vi "StandardInit.vi"(1 "Incoming Handle":i32) -> (0 "Outgoing Handle":i32)   [LabVIEW 2011]
uses:
  Program Files (x86)/Gelles Lab Software/Madlib.dll
panel:
  out "Serial #":i32
  out "Aux axis":bool
  out "Aux Calibration":dbl format="%.3f"
  out "Z axis":bool
  out "Z Calibration":dbl format="%.3f"
  out "Y axis":bool
  out "Y Calibration":dbl format="%.3f"
  out "X axis":bool
  out "X Calibration":dbl caption="Calibration (um)" format="%.3f"
  out "DAC Freq (ms)":dbl format="%.4f"
  out "ADC Freq (ms)":dbl format="%.4f"
  out "Dll Revision":i16
  out "Dll Version":i16
  out "ADC resolution (bits)":i16
  out "DAC resolution (bits)":i16
  out "Product ID (in hex)":string
  out "Firmware Version":i16
  out "Firmware Profile":i16
  # "This VI implements an initialization sequence for use with \na single Nano-Drive."
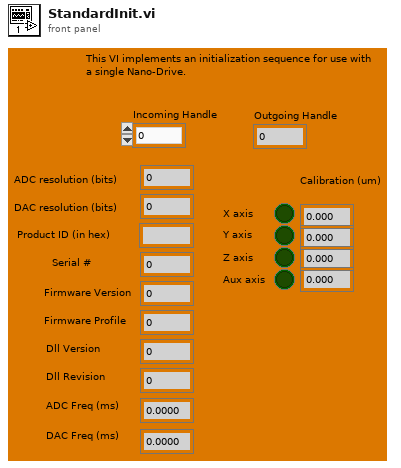
[diagram p1: front panel]
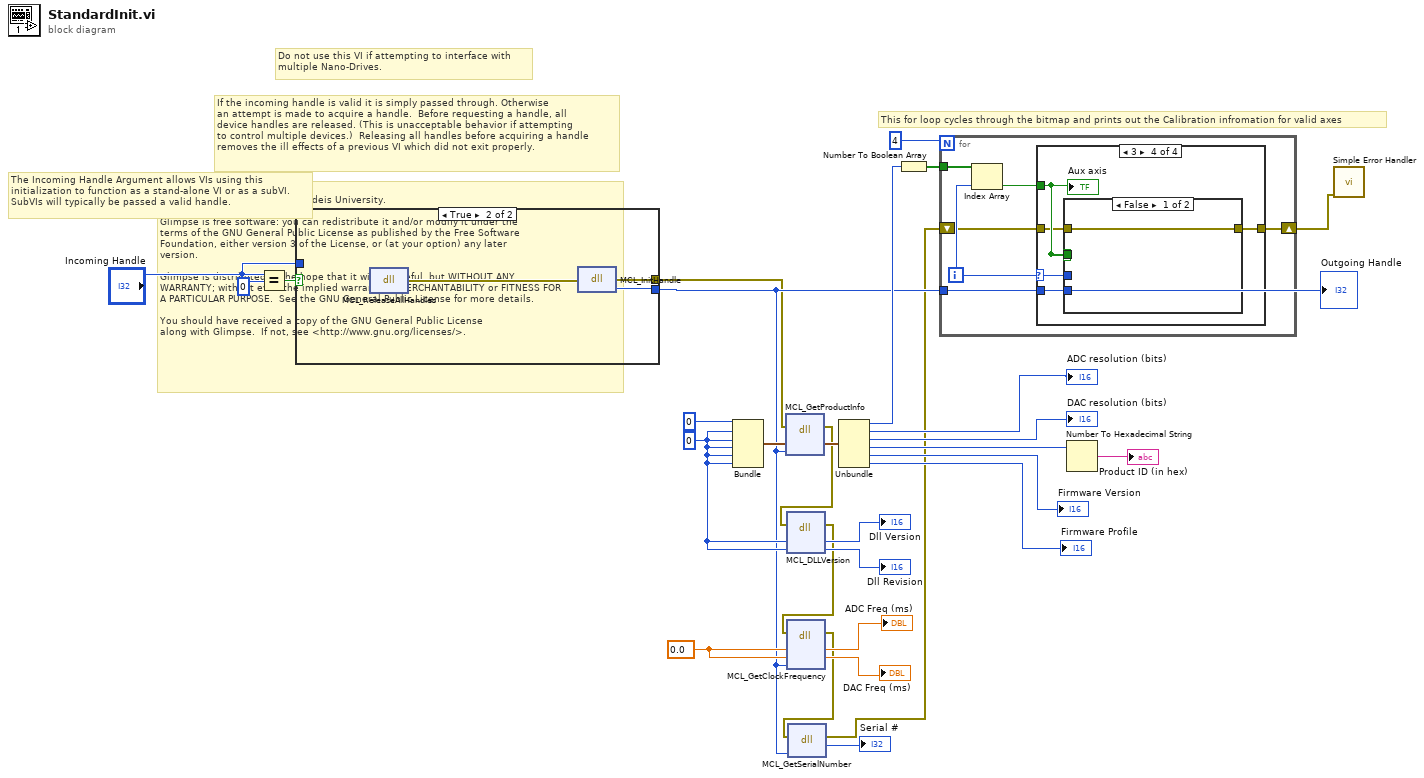
[diagram p0: block diagram]
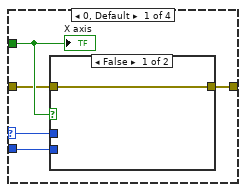
[diagram p2: hidden frame]
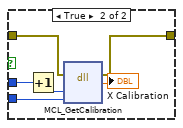
[diagram p3: hidden frame]
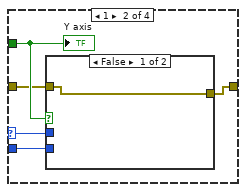
[diagram p4: hidden frame]
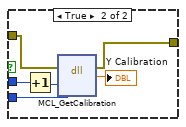
[diagram p5: hidden frame]
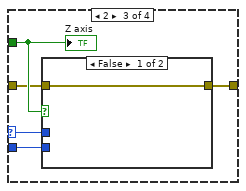
[diagram p6: hidden frame]
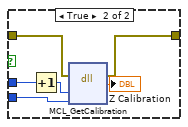
[diagram p7: hidden frame]
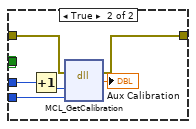
[diagram p8: hidden frame]
diagram:
  w14 = 0.0
  w17 = i16 0
  # "This file is part of Glimpse. \nCopyright 2014 Jeff Gelles, Brandeis University.    \n\nGlimpse is free software: you can redistribute it and/or modify it under the \nterms of the GNU General Public License as published by the Free Software \nFoundation, either version 3 of the License, or (at your option) any later \nversion.\n\nGlimpse is distributed in the hope that it will be useful, but WITHOUT ANY \nWARRANTY; without even the implied warranty of MERCHANTABILITY or FITNESS FOR \nA PARTICULAR PURPOSE.  See the GNU General Public License for more details.\n\nYou should have received a copy of the GNU General Public License\nalong with Glimpse.  If not, see <http://www.gnu.org/licenses/>."
  # "This for loop cycles through the bitmap and prints out the Calibration infromation for valid axes"
  # "The Incoming Handle Argument allows VIs using this\ninitialization to function as a stand-alone VI or as a subVI.\nSubVIs will typically be passed a valid handle."
  # "Do not use this VI if attempting to interface with\nmultiple Nano-Drives."
  # "If the incoming handle is valid it is simply passed through. Otherwise\nan attempt is made to acquire a handle.  Before requesting a handle, all\ndevice handles are released. (This is unacceptable behavior if attempting\nto control multiple devices.)  Releasing all handles before acquiring a handle\nremoves the ill effects of a previous VI which did not exit properly."
  n1 = Equal?(x="Incoming Handle", y=0) -> (x = y?=w28:bool)
  n2 = case shown="True" w28 {
    tunnel: [w30 w33] -> w7
    tunnel: "Incoming Handle" -> [w30 _]
    tunnel: [_ w31] -> w6
    frame False {
    }
    frame True {
      n3 = dll-call lib="C:/Program Files (x86)/Gelles Lab Software/MADLib.dll" fn="MCL_ReleaseAllHandles"() -> (error out=w32:errorcluster)  [unwired: 4 in, 1 out]
      n4 = dll-call lib="C:/Program Files (x86)/Gelles Lab Software/MADLib.dll" fn="MCL_InitHandle"(error in=w32) -> (error out=w31:errorcluster, "return type"=w33:i32)  [unwired: 2 in, 1 out]
    }
  }
  "Outgoing Handle" <- w7
  n5 = Bundle(u8 0, w17, w17, w17, w17, w17) -> (w25:cluster{u8, i16, i16, i16, i16, i16})  [unwired: 1 in]
  n6 = dll-call lib="C:/Program Files (x86)/Gelles Lab Software/MADLib.dll" fn="MCL_GetProductInfo"(error in=w6, w25, "handle"=w7) -> (error out=w5:errorcluster, w24:cluster{u8, i16, i16, i16, i16, i16})  [unwired: 4 in, 1 out]
  n7 = dll-call lib="C:/Program Files (x86)/Gelles Lab Software/MADLib.dll" fn="MCL_DLLVersion"(error in=w5, "version"=w17, "revision"=w17) -> (error out=w4:errorcluster, "version"=→"Dll Version":i16, "revision"=→"Dll Revision":i16)  [unwired: 3 in, 1 out]
  n8 = dll-call lib="C:/Program Files (x86)/Gelles Lab Software/MADLib.dll" fn="MCL_GetClockFrequency"(error in=w4, "ADC freq"=w14, "DAC freq"=w14, "handle"=w7) -> (error out=w3:errorcluster, "ADC freq"=→"ADC Freq (ms)":dbl, "DAC freq"=→"DAC Freq (ms)":dbl)  [unwired: 4 in, 1 out]
  n9 = dll-call lib="C:/Program Files (x86)/Gelles Lab Software/MADLib.dll" fn="MCL_GetSerialNumber"(error in=w3, "handle"=w7) -> (error out=w2:errorcluster, →"Serial #":i32)  [unwired: 3 in, 1 out]
  n10 = Unbundle(w24) -> (w11:u8, →"ADC resolution (bits)":i16, →"DAC resolution (bits)":i16, w23:i16, →"Firmware Version":i16, →"Firmware Profile":i16)
  n11 = Number To Boolean Array(number=w11) -> (Boolean array=w10:bool[])
  n12 = for {
    N: 4 -> [_]
    tunnel: w10 -> [w39]
    tunnel: w7 -> [w36]
    shift-right: [w34] -> w1
    shift-left: w2 -> [w35]
    i -> [w38]
    n13 = Index Array(array=w39, index=w38) -> (element=w37:bool)
    n14 = case shown="3" w38 {
      selector: w38 -> [w44 w56 w68 w80]
      tunnel: w37 -> [w43 w55 w67 w79]
      tunnel: w36 -> [w42 w54 w66 w78]
      tunnel: w35 -> [w41 w53 w65 w77]
      tunnel: [w40 w52 w64 w76] -> w34
      frame 0, Default {
        n15 = case shown="False" w43 {
          tunnel: w44 -> [_ w51]
          tunnel: w42 -> [_ w48]
          tunnel: w41 -> [w45 w47]
          tunnel: [w45 w46] -> w40
          frame False {
          }
          frame True {
            n16 = Increment(x=w51) -> (x+1=w49:i32)
            n17 = dll-call lib="C:/Program Files (x86)/Gelles Lab Software/MADLib.dll" fn="MCL_GetCalibration"(error in=w47, "axis"=w49, "handle"=w48) -> (error out=w46:errorcluster, →"X Calibration":dbl)  [unwired: 4 in, 1 out]
          }
        }
        "X axis" <- w43
      }
      frame 1 {
        n18 = case shown="False" w55 {
          tunnel: w56 -> [_ w63]
          tunnel: w54 -> [_ w61]
          tunnel: w53 -> [w57 w59]
          tunnel: [w57 w58] -> w52
          frame False {
          }
          frame True {
            n19 = Increment(x=w63) -> (x+1=w62:i32)
            n20 = dll-call lib="C:/Program Files (x86)/Gelles Lab Software/MADLib.dll" fn="MCL_GetCalibration"(error in=w59, "axis"=w62, "handle"=w61) -> (error out=w58:errorcluster, →"Y Calibration":dbl)  [unwired: 4 in, 1 out]
          }
        }
        "Y axis" <- w55
      }
      frame 2 {
        n21 = case shown="False" w67 {
          tunnel: w68 -> [_ w75]
          tunnel: w66 -> [_ w73]
          tunnel: w65 -> [w69 w71]
          tunnel: [w69 w70] -> w64
          frame False {
          }
          frame True {
            n22 = Increment(x=w75) -> (x+1=w72:i32)
            n23 = dll-call lib="C:/Program Files (x86)/Gelles Lab Software/MADLib.dll" fn="MCL_GetCalibration"(error in=w71, "axis"=w72, "handle"=w73) -> (error out=w70:errorcluster, →"Z Calibration":dbl)  [unwired: 4 in, 1 out]
          }
        }
        "Z axis" <- w67
      }
      frame 3 {
        n24 = case shown="False" w79 {
          tunnel: w80 -> [_ w87]
          tunnel: w79 -> [_ _]
          tunnel: w78 -> [_ w84]
          tunnel: w77 -> [w81 w83]
          tunnel: [w81 w82] -> w76
          frame False {
          }
          frame True {
            n25 = Increment(x=w87) -> (x+1=w85:i32)
            n26 = dll-call lib="C:/Program Files (x86)/Gelles Lab Software/MADLib.dll" fn="MCL_GetCalibration"(error in=w83, "axis"=w85, "handle"=w84) -> (error out=w82:errorcluster, →"Aux Calibration":dbl)  [unwired: 4 in, 1 out]
          }
        }
        "Aux axis" <- w79
      }
    }
  }
  n27 = Number To Hexadecimal String(2:w23) -> (0:→"Product ID (in hex)":string)  [unwired: 1 in]
  n28 = call <vilib>:"Simple Error Handler.vi"("error in (no error)"=w1) -> ()  [unwired: 4 in, 5 out]
